vi "LINX - PmodJSTK.vi"() -> ()   [LabVIEW 2014, in "LMH-LINX.lvlib"]
doc: "PmodJSTK\n\nThis example demonstrates how to read joystick position, button pushes, and write LED settings to the PmodJSTK. \n\nInstructions:\n1. Select the COM Port associated with the LINX device\n2. Select the SPI Channel that the Pmod is connected to.\n3. Select the CS Channel that the Pmod is connected to.\n4. Use the control to select the LED configuration\n5. Click the Run Arrow."
uses:
  vi.lib/MakerHub/LINX/LMH-LINX.lvlib
  vi.lib/MakerHub/LINX/Public/Utilities/Open Serial.vi
  vi.lib/MakerHub/LINX/Public/Sensors/Pmods/JSTK/PmodJSTK.lvlib
panel:
  in  "Stop Button":bool
  out "Y - Axis":string
  out "X - Axis":string
  out "Buttons":u8
  in  "CS Channel":u8
  in  "SPI Channel (0)":u8
  in  "LEDs":enum16{"None", "LD1", "LD2", "Both"}(ring)=enum."LD2"
  in  "Serial Port":refnum<visa-resource-name>="N/A"
  # "PmodJSTK Button Layout"
  # "Joystick Button = Bit 1\nButton 1 = Bit 2\nButton 2 = Bit 3"
  # "Combinations"
  # "Bit 3 | Bit 2 | Bit 1"
  # "Result"
  # "0        0         0\n0        0         1\n0        1         0\n0        1         1\n1        0         0\n1        0         1\n1        1         0\n1        1         1"
  # "0\n1\n2\n3\n4\n5\n6\n7"
  # "PmodJSTK\n\nThis example demonstrates how to read joystick position, button pushes, and write LED settings to the PmodJSTK. \n\nInstructions:\n1. Select the COM Port associated with the LINX device\n2. Select the SPI Channel that the Pmod is connected to.\n3. Select the CS Channel that the Pmod is connected to.\n4. Use the control to select the LED configuration\n5. Click the Run Arrow."
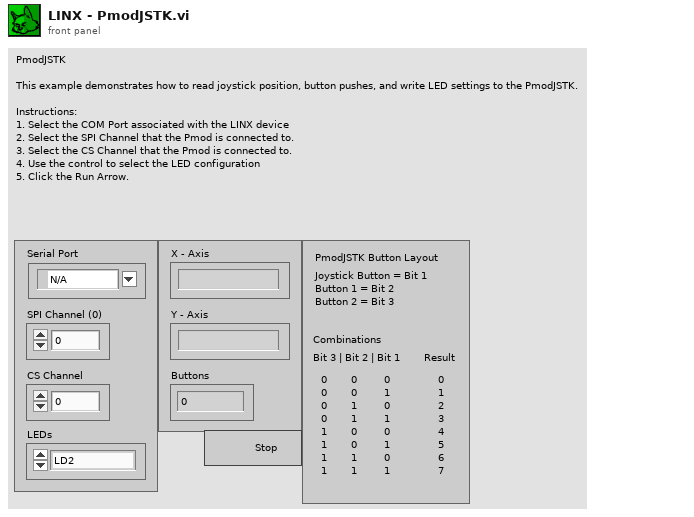
[diagram p1: front panel]
types:
  T1 = typedef "LMH-LINX.lvlib/LINX Ref.ctl" = cluster{"IO":T2, "Interface":T3, "LINX Device Config":T4}
  T2 = typedef "LMH-LINX.lvlib/Platform.ctl" = enum16{"Remote", "Local"}
  T3 = typedef "LMH-LINX.lvlib/Interface.ctl" = enum16{"Serial", "TCP"}
  T4 = typedef "LMH-LINX.lvlib/Device.lvlib/LINX Device Config.ctl" = cluster{"Interface":T3, "COM Port":refnum<visa-resource-name>, "TCP Configuration":T5, "Device Family":u8, "Device ID":u8, "Device Name":string, "TCP Ref":refnum<k5>, "Channels":T6}
  T5 = typedef "LMH-LINX.lvlib/Device.lvlib/TCP Config.ctl" = cluster{"IP Address":string, "Port":u16}
  T6 = typedef "LMH-LINX.lvlib/Channels.ctl" = cluster{"DI":u8[], "DO":u8[], "AI":u8[], "AO":u8[], "PWM":u8[], "QE":u8[], "UART":u8[], "I2C 2":u8[], "SPI":u8[], "CAN":u8[], "Servo":u8[], "AI Ref (V)":dbl, "AI Resolution (Bits)":u8, "AO Ref (V)":dbl, "AO Resolution (Bits)":u8}
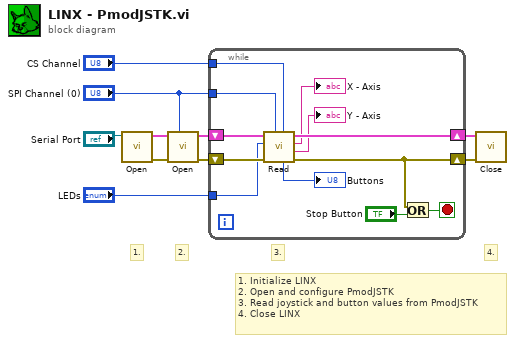
[diagram p0: block diagram]
diagram:
  # "1. Initialize LINX\n2. Open and configure PmodJSTK\n3. Read joystick and button values from PmodJSTK\n4. Close LINX"
  # "4."
  # "3."
  # "2."
  # "1."
  n1 = call-poly "Open.vi"("Serial Port"="Serial Port") -> ("Error Out"=w9:errorcluster, "LINX Resource"=w10:T1)  [unwired: 8 in, 1 out]
  n2 = call "Open.vi"("SPI Channel (0)"="SPI Channel (0)", "Error In"=w9, "LINX Resource"=w10) -> ("Error Out"=w6:errorcluster, "LINX Resource"=w7:T1)  [unwired: 7 in]
  n3 = while {
    tunnel: "LEDs" -> [w20]
    tunnel: "SPI Channel (0)" -> [w19]
    tunnel: "CS Channel" -> [w18]
    shift-right: [w16] -> w3
    shift-left: w7 -> [w22]
    shift-right: [w13] -> w2
    shift-left: w6 -> [w21]
    stop <- w12 stop-if-true
    n4 = call "Read.vi"("CS Channel"=w18, "SPI Channel (0)"=w19, "Error In"=w21, "LEDs"=w20, "LINX Resource"=w22) -> ("Error Out"=w13:errorcluster, "Y - Axis"=→"Y - Axis":string, "X - Axis"=→"X - Axis":string, "LINX Resource"=w16:T1, "Buttons"=→"Buttons":u8)  [unwired: 2 in]
    n5 = Or(x=w13, y="Stop Button") -> (x .or. y?=w12:bool)
  }
  n6 = call "Close.vi"("Error In"=w2, "LINX Resource"=w3) -> ()  [unwired: 9 in, 1 out]
